vi "StringToNumber4.vi"(8 "string 4":string, 9 "string 3":string, 10 "string 2":string, 11 "string":string) -> (0 "Numeric 4":dbl, 1 "Numeric 3":dbl, 2 "Numeric 2":dbl, 3 "Numeric":dbl)   [LabVIEW 2012]
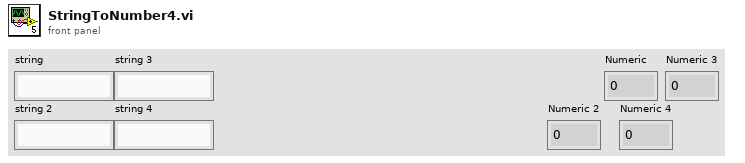
[diagram p1: front panel]
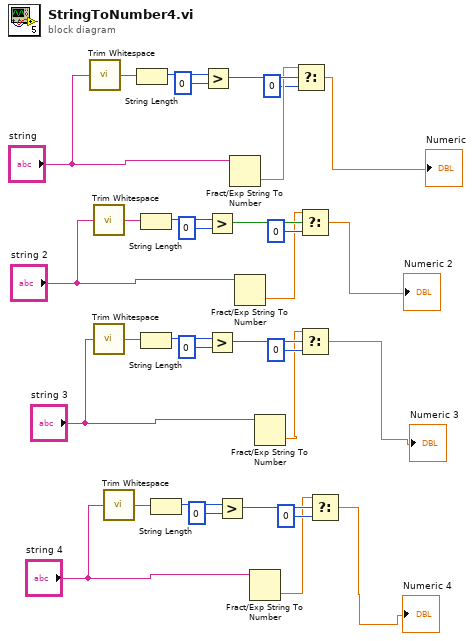
[diagram p0: block diagram]
diagram:
  n1 = call <vilib>:"Trim Whitespace.vi"("string"="string") -> ("trimmed string"=w30:string)  [unwired: 1 in]
  n2 = call <vilib>:"Trim Whitespace.vi"("string"="string 2") -> ("trimmed string"=w22:string)  [unwired: 1 in]
  n3 = call <vilib>:"Trim Whitespace.vi"("string"="string 3") -> ("trimmed string"=w14:string)  [unwired: 1 in]
  n4 = call <vilib>:"Trim Whitespace.vi"("string"="string 4") -> ("trimmed string"=w6:string)  [unwired: 1 in]
  n5 = String Length(string=w30) -> (length=w32:i32)
  n6 = String Length(string=w22) -> (length=w24:i32)
  n7 = String Length(string=w14) -> (length=w16:i32)
  n8 = String Length(string=w6) -> (length=w8:i32)
  n9 = Greater?(x=w32, y=0) -> (0:w28:bool)
  n10 = Greater?(x=w24, y=0) -> (0:w21:bool)
  n11 = Greater?(x=w16, y=0) -> (0:w13:bool)
  n12 = Greater?(x=w8, y=0) -> (0:w5:bool)
  n13 = Fract/Exp String To Number(string="string") -> (number=w27:dbl)  [unwired: 3 in, 1 out]
  n14 = Fract/Exp String To Number(string="string 2") -> (number=w18:dbl)  [unwired: 3 in, 1 out]
  n15 = Fract/Exp String To Number(string="string 4") -> (number=w2:dbl)  [unwired: 3 in, 1 out]
  n16 = Fract/Exp String To Number(string="string 3") -> (number=w10:dbl)  [unwired: 3 in, 1 out]
  n17 = Select(t=w27, s=w28, f=0) -> (s? t:f=→"Numeric":dbl)
  n18 = Select(t=w18, s=w21, f=0) -> (s? t:f=→"Numeric 2":dbl)
  n19 = Select(t=w10, s=w13, f=0) -> (s? t:f=→"Numeric 3":dbl)
  n20 = Select(t=w2, s=w5, f=0) -> (s? t:f=→"Numeric 4":dbl)
